vi "Internal Start Loop.vi"(8 "error in (no error)":errorcluster, 11 "navX Device":T1={"Interface"={"Protocol"=enum."SERIAL", "Update Rate (4Hz-60Hz)"=4, "navX Open TypeDef"=variant}, "Notify Packet"=refnum, "Loop VI Refnum"=refnum} {"Interface"."Update Rate (4Hz-60Hz)" min=4 max=60 step=1}) -> (0 "error out":errorcluster, 3 "navX Device":T1={"Interface"={"Protocol"=enum."SERIAL", "Update Rate (4Hz-60Hz)"=4, "navX Open TypeDef"=variant}, "Notify Packet"=refnum, "Loop VI Refnum"=refnum} {"Interface"."Update Rate (4Hz-60Hz)" min=4 max=60 step=1})   [LabVIEW 2014, in "navX Library v2.lvlib"]
uses:
  navX Library v2.lvlib
  TypeDefs/navX Device TypeDef.ctl
  TypeDefs/navX Protocol TypeDef.ctl
  TypeDefs/navX Notify Packet TypeDef.ctl
  TypeDefs/navX Action TypeDef.ctl
  Processing Loop.vi
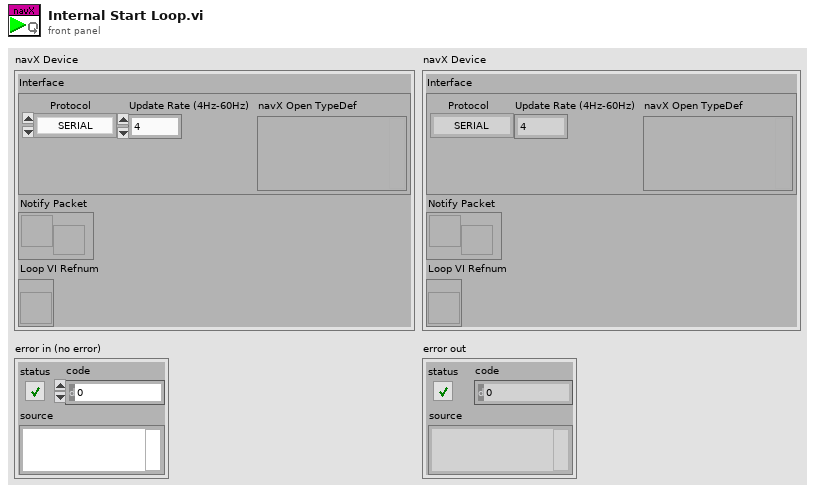
[diagram p1: front panel]
types:
  T1 = typedef "navX Library v2.lvlib/navX Device TypeDef.ctl" = cluster{"Interface":cluster{"Protocol":T2, "Update Rate (4Hz-60Hz)":u8, "navX Open TypeDef":variant}, "Notify Packet":refnum<notifier>, "Loop VI Refnum":refnum<vi>}
  T2 = typedef "navX Library v2.lvlib/navX Protocol TypeDef.ctl" = enum16{"SERIAL", "I2C", "SPI"}
  T3 = typedef "navX Library v2.lvlib/navX Notify Packet TypeDef.ctl" = cluster{"navX Action":T4, "Data":variant}
  T4 = typedef "navX Library v2.lvlib/navX Action TypeDef.ctl" = enum16{"None", "Halt", "Reboot Detected", "Zero-Yaw"}
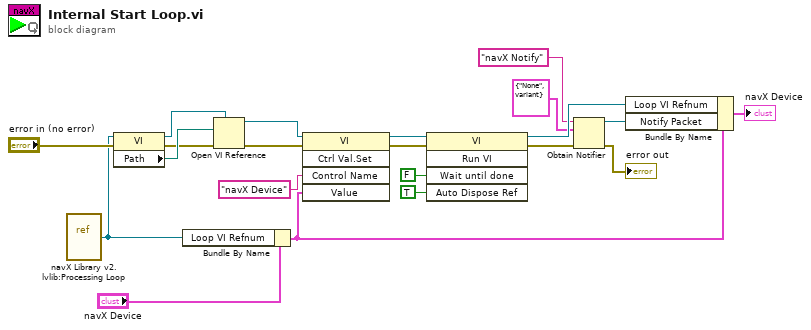
[diagram p0: block diagram]
diagram:
  n1 = vi-ref "navX Library v2.lvlib:Processing Loop.vi"() -> (w19:refnum<vi>)
  n2 = property class="VI"(reference=w19, error in="error in (no error)") -> (reference out=w16:refnum<vi>, error out=w17:errorcluster, "Path"=w18:path)
  n3 = Bundle By Name(cluster="navX Device", "Loop VI Refnum"=w19) -> (w9:T1)
  n4 = Open VI Reference(type specifier VI Refnum (for type only)=w16, vi path=w18, error in (no error)=w17) -> (vi reference=w6:refnum<vi>, error out=w15:errorcluster)  [unwired: 3 in]
  n5 = invoke class="VI" method="Ctrl Val.Set"(reference=w6, error in=w15, "Control Name"="navX Device", "Value"=w9) -> (reference out=w13:refnum<vi>, error out=w12:errorcluster)  [unwired: 1 in, 3 out]
  n6 = invoke class="VI" method="Run VI"(reference=w13, error in=w12, "Wait until done"=FALSE ("Wait Until Done"), "Auto Dispose Ref"=TRUE ("Auto Dispose Reference")) -> (reference out=w8:refnum<vi>, error out=w2:errorcluster)  [unwired: 1 in, 3 out]
  n7 = Obtain Notifier(name (unnamed)="navX Notify", notification data type=T3 {"navX Action"=enum."None", "Data"=variant} ("navX Notify Packet"), error in (no error)=w2) -> (notifier out=w5:refnum<notifier>, error out=→"error out":errorcluster)  [unwired: 1 in, 1 out]
  n8 = Bundle By Name(cluster=w9, "Loop VI Refnum"=w8, "Notify Packet"=w5) -> (→"navX Device":T1)
